vi "LV INIT SPECTRUM.vi"(0 "min":u32, 1 "max":u32=65535, 2 "limitmode":string(combo)="freerun", 3 "limit":u32, 5 "rebin":u32, 7 "Spectrum name":string, 9 "Handle In":T2) -> (10 "Handle Out":T1)   [LabVIEW 2021]
uses:
  SciSDK_Labview.lvlib
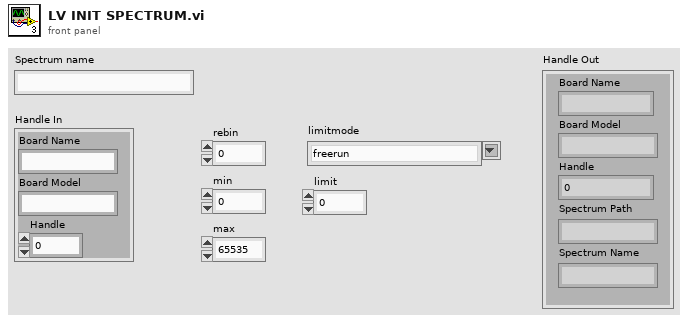
[diagram p1: front panel]
types:
  T1 = cluster{"Board Name":string, "Board Model":string, "Handle":u64, "Spectrum Path":string, "Spectrum Name":string}
  T2 = cluster{"Board Name":string, "Board Model":string, "Handle":u64}
  T3 = cluster{"Board Name":string, "Board Model":string, "Handle":u64, string, "Spectrum name":string}
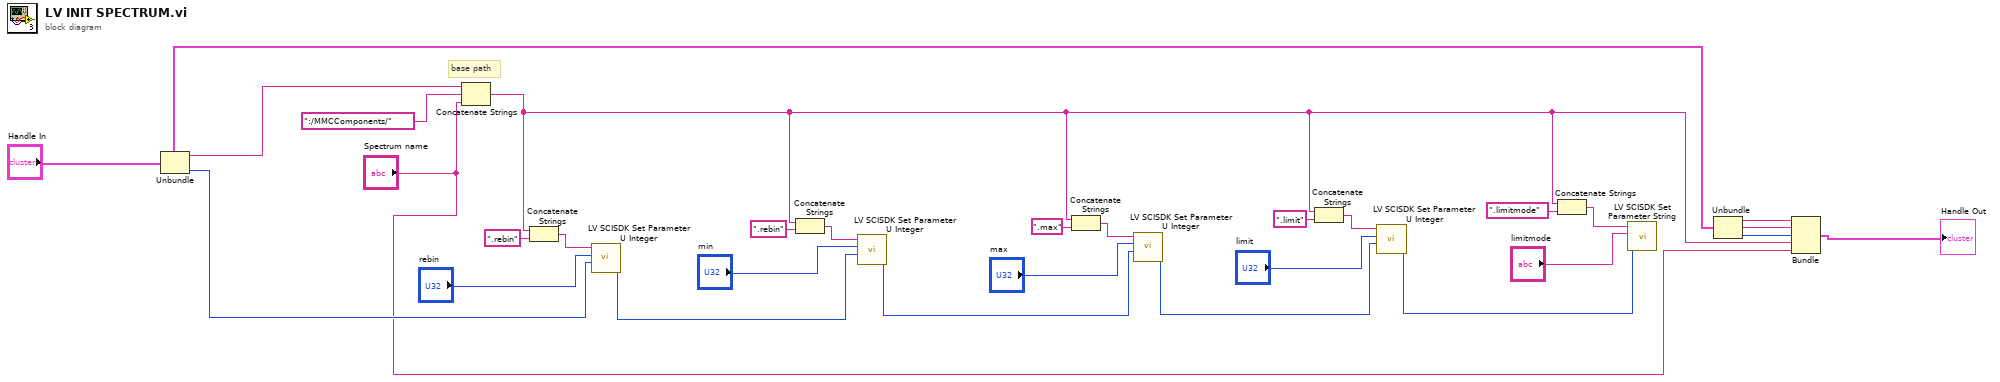
[diagram p0: block diagram]
diagram:
  # "base path"
  n1 = Unbundle("Handle In") -> ("Board Name"=w28:string, "Handle"=w24:u64)  [unwired: 1 out]
  n2 = Concatenate Strings(w28, ":/MMCComponents/" ("string"), "Spectrum name") -> (w2:string)
  n3 = Concatenate Strings(w2, ".rebin" ("string")) -> (w26:string)
  n4 = call "LV SCISDK Set Parameter U Integer.vi"("handle"=w24, "value"="rebin", "Path"=w26) -> ("handle out"=w17:u64)  [unwired: 6 in, 2 out]
  n5 = Concatenate Strings(w2, ".rebin" ("string")) -> (w22:string)
  n6 = call "LV SCISDK Set Parameter U Integer.vi"("handle"=w17, "value"="min", "Path"=w22) -> ("handle out"=w15:u64)  [unwired: 6 in, 2 out]
  n7 = Concatenate Strings(w2, ".max" ("string")) -> (w20:string)
  n8 = call "LV SCISDK Set Parameter U Integer.vi"("handle"=w15, "value"="max", "Path"=w20) -> ("handle out"=w13:u64)  [unwired: 6 in, 2 out]
  n9 = Concatenate Strings(w2, ".limit" ("string")) -> (w18:string)
  n10 = call "LV SCISDK Set Parameter U Integer.vi"("handle"=w13, "value"="limit", "Path"=w18) -> ("handle out"=w11:u64)  [unwired: 6 in, 2 out]
  n11 = Concatenate Strings(w2, ".limitmode" ("string")) -> (w8:string)
  n12 = call "LV SCISDK Set Parameter String.vi"("handle"=w11, "value"="limitmode", "Path"=w8) -> ()  [unwired: 6 in, 3 out]
  n13 = Unbundle("Handle In") -> ("Board Name"=w6:string, "Board Model"=w5:string, "Handle"=w4:u64)
  n14 = Bundle("Board Name"=w6, "Board Model"=w5, "Handle"=w4, w2, "Spectrum name"="Spectrum name") -> (→"Handle Out":T3)  [unwired: 1 in]
